vi "Prepare to Load New File.vi"(7 "AppData In":T1, 10 "Data Path":path, 11 "AppState In":T2) -> (3 "AppState Out":T2, 5 "AppData Out":T1)   [LabVIEW 2019]
uses:
  TypeDef/App State.ctl
  TypeDef/App Data.ctl
  TypeDef/File Type.ctl
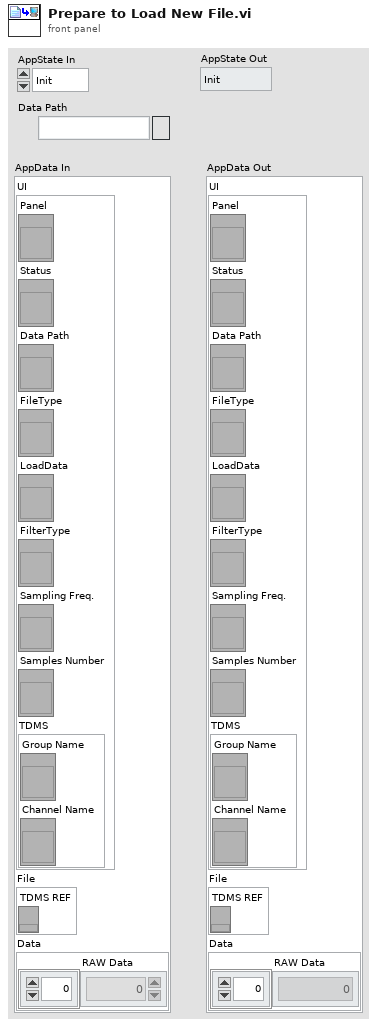
[diagram p1: front panel]
types:
  T1 = typedef "App Data.ctl" = cluster{"UI":cluster{"Panel":refnum<vi>, "Status":refnum<vi>, "Data Path":refnum<vi>, "FileType":refnum<vi>, "LoadData":refnum<vi>, "FilterType":refnum<vi>, "Sampling Freq.":refnum<vi>, "Samples Number":refnum<vi>, "TDMS":cluster{"Group Name":refnum<vi>, "Channel Name":refnum<vi>}}, "File":cluster{"TDMS REF":refnum<k34>}, "Data":cluster{"RAW Data":dbl[]}}
  T2 = typedef "App State.ctl" = enum16{"Init", "LoadFile", "LoadDataFromFile", "RunFilter", "GenerateRaport", "Exit"}
  T3 = typedef "File Type.ctl" = enum32{"TDMS", "CSV"}
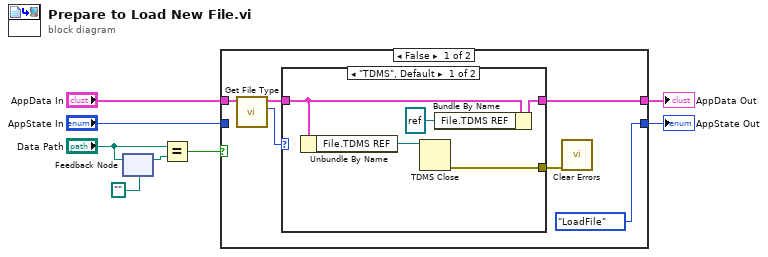
[diagram p0: block diagram]
diagram:
  n1 = feedback #1(path "") -> (w7:path)
  n2 = feedback-in #1("Data Path") -> ()
  n3 = Equal?(x="Data Path", y=w7) -> (x = y?=w2:bool)
  n4 = case shown="False" w2 {
    tunnel: "AppData In" -> [w13 w22]
    tunnel: [w11 w22] -> w5
    tunnel: "AppState In" -> [_ w21]
    tunnel: [App_State."LoadFile" ("f") w21] -> w3
    frame False {
      n5 = call "Get File Type.vi"("App Data In"=w13) -> ("FileType"=w12:T3, "App Data Out"=w10:T1)  [unwired: 9 in]
      n6 = case shown="\"TDMS\", Default" w12 {
        tunnel: [w16 w20] -> w11
        tunnel: w10 -> [w19 w20]
        tunnel: [w17 _] -> w9
        frame "TDMS", Default {
          n7 = Unbundle By Name(w19) -> ("File.TDMS REF"=w18:refnum<k34>)
          n8 = TDMS Close(11:w18) -> (0:w17:errorcluster)  [unwired: 1 in, 1 out]
          n9 = Bundle By Name(cluster=w19, "File.TDMS REF"=refnum<k34> refnum) -> (w16:T1)
        }
        frame "CSV" {
        }
      }
      n10 = call <vilib>:"Clear Errors.vi"("error in (no error)"=w9) -> ()  [unwired: 5 in, 2 out]
    }
    frame True {
    }
  }
  "AppState Out" <- w3
  "AppData Out" <- w5
